vi "ATS_Close.vi"(8 "error in (no error)":errorcluster, 11 "Handle":u32) -> ()   [LabVIEW 2016]
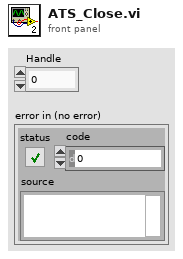
[diagram p1: front panel]
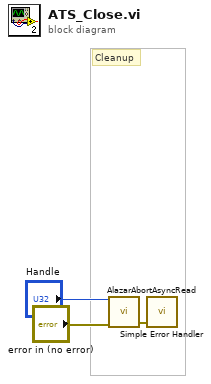
[diagram p0: block diagram]
diagram:
  # "Cleanup"
  n1 = call "AlazarAbortAsyncRead.vi"("Handle"="Handle", "error in (no error)"="error in (no error)") -> ("error out"=w1:errorcluster)  [unwired: 2 out]
  n2 = call <vilib>:"Simple Error Handler.vi"("error in (no error)"=w1) -> ()  [unwired: 4 in, 5 out]
